vi "Inspect Tell.vi"(4 "Unified Actor Alias":string, 10 "Msg DVR":refnum<data-value>, 11 "Base Actor in":refnum<class "Base Actor.lvclass">) -> (3 "Base Actor out":refnum<class "Base Actor.lvclass">)   [LabVIEW 2020, in "jettl.lvlib" / "BaseActor.lvlib" / "Base Actor.lvclass"]
uses:
  Base Actor.lvclass
  Base Actor.lvclass/Base Actor.ctl
  ActorRelation.ctl
  jettl.lvlib
  MessageMetadata.ctl
  Message/Message.lvclass
  Message.ctl
  ActorLifetime.ctl
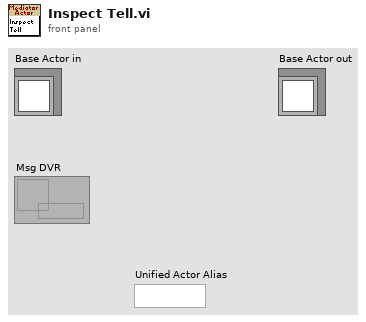
[diagram p1: front panel]
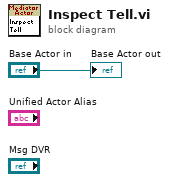
[diagram p0: block diagram]
diagram:
  "Base Actor out" <- "Base Actor in"
